vi "Read Test Finder.vi"(8 "error in (no error)":errorcluster, 11 "Test Finder In":refnum<class "Finder Test.lvclass">) -> (0 "error out":errorcluster, 2 "Test Finder.lvclass":refnum<class "Test Finder.lvclass">, 3 "Test Finder Out":refnum<class "Finder Test.lvclass">)   [LabVIEW 2020, in "LUnit Tests.lvlib" / "Finder Test.lvclass"]
uses:
  Finder Test.lvclass
  Finder Test.lvclass/Finder Test.ctl
  source/Framework/Helper Classes/Test Finder/Test Finder.lvclass
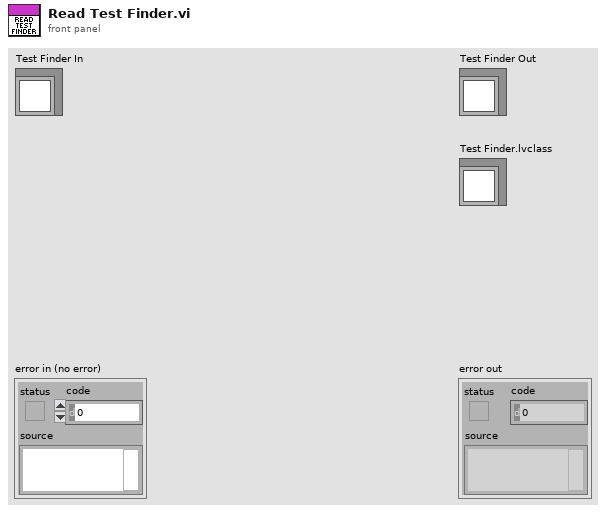
[diagram p1: front panel]
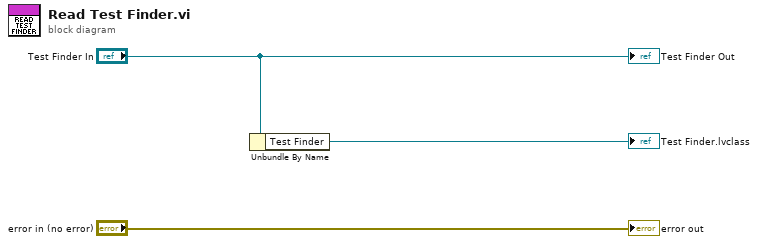
[diagram p0: block diagram]
diagram:
  n1 = Unbundle By Name("Test Finder In") -> ("Test Finder"=→"Test Finder.lvclass":refnum<class "Test Finder.lvclass">)
  "error out" <- "error in (no error)"
  "Test Finder Out" <- "Test Finder In"
